vi "Convert CAN Frame to String.vi"(8 "error in":errorcluster, 11 "element":T1 {"payload" format="%x"; "timestamp" format="%<%.7X\n%x>T"; "type" items=["CAN Data"=0, "CAN Remote"=1, "CAN Bus Error"=2, "CAN 2.0 Data"=8, "CAN FD Data"=16, "CAN FD+BRS Data"=24, "J1939 Data"=192, "Delay"=224, "Log Trigger"=225, "Start Trigger"=226]; "identifier" format="%x"}) -> (0 "error out":errorcluster, 3 "String":string)   [LabVIEW 2019, in "J1939 Workspace Shared.lvlib"]
uses:
  J1939 Workspace Shared.lvlib
  <vilib>/xnet/xnet.llb/XNET Frame CAN.ctl
  <vilib>/xnet/xnet.llb/XNET Frame Type CAN.ctl
  <vilib>/Utility/error.llb/DialogType.ctl
  Addon/Support Libraries/J1939 Utilities/SubVIs/Convert CAN Arb ID to J1939 ID.vi
  Addon/Support Libraries/J1939 Utilities/J1939 Utilities.lvlib
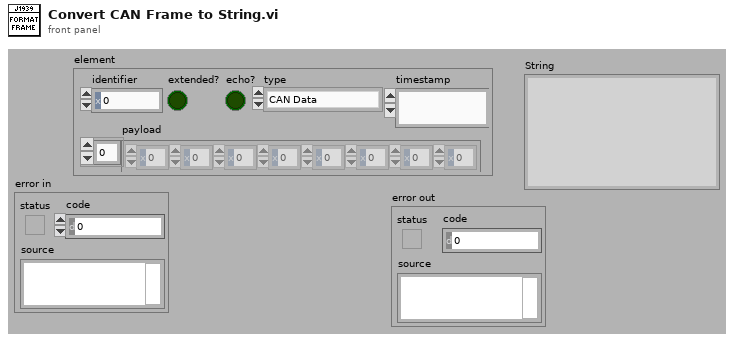
[diagram p1: front panel]
types:
  T1 = typedef "XNET Frame CAN.ctl" = cluster{"timestamp":timestamp, "payload":u8[], "identifier":u32, "type":T2, "extended?":bool, "echo?":bool}
  T2 = typedef "XNET Frame Type CAN.ctl" = u8
  T3 = typedef "DialogType.ctl" = u16
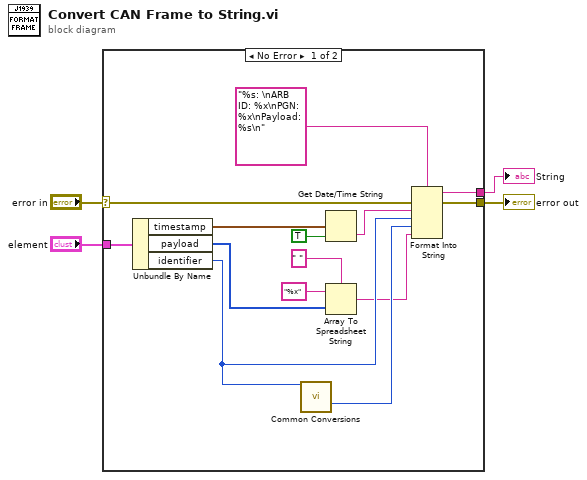
[diagram p0: block diagram]
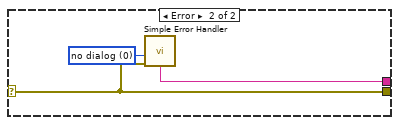
[diagram p2: hidden frame]
diagram:
  n1 = case shown="No Error" "error in" {
    selector: "error in" -> [w5 w21]
    tunnel: "element" -> [w16 _]
    tunnel: [w11 w19] -> w3
    tunnel: [w6 w21] -> w2
    frame No Error {
      n2 = Unbundle By Name(w16) -> ("timestamp"=w17:timestamp, "payload"=w9:u8[], "identifier"=w13:u32)
      n3 = call-poly "Common Conversions.vi"("Arb ID"=w13) -> ("PGN"=w12:u32)  [unwired: 14 out]
      n4 = Get Date/Time String(seconds (now)=w17, want seconds? (F)=TRUE) -> (time string=w14:string)  [unwired: 1 in, 1 out]
      n5 = Array To Spreadsheet String(delimiter (Tab)=" ", array=w9, 3:"%x" ("format string")) -> (spreadsheet string=w7:string)
      n6 = Format Into String(format string="%s: \nARB ID: %x\nPGN: %x\nPayload: %s\n", error in=w5, w14, w13, w12, w7) -> (resulting string=w11:string, error out=w6:errorcluster)  [unwired: 1 in]
    }
    frame Error {
      w20 = T3 0 items=["no dialog", "OK message", "continue or stop message", "OK message + warnings", "continue/stop + warnings"] ("type of dialog (OK msg:1)")
      n7 = call <vilib>:"Simple Error Handler.vi"("type of dialog (OK msg:1)"=w20, "error in (no error)"=w21) -> ("message"=w19:string)  [unwired: 3 in, 4 out]
    }
  }
  "String" <- w3
  "error out" <- w2
